vi "REV2mDistanceSensorRefNum Registry Set.vi"(8 "error in (no error)":errorcluster, 9 "Test Mode Only":bool, 10 "refnum name":string="REV2m", 11 "REV2mDistanceSensorsArray":T1={"Automatic Enabled"=TRUE, "Sensors[]"=[]}) -> (0 "error out":errorcluster, 3 "REV2mDistanceSensorsArray Out":T1={"Automatic Enabled"=TRUE, "Sensors[]"=[]})   [LabVIEW 2019, in "DistanceSensorDriver.lvlib"]
uses:
  DistanceSensorDriver.lvlib
  Typedef/Rev2mDistanceSensorsArray.ctl
  Typedef/REV2mDistanceSensorDevRef.ctl
  Typedef/Ports.ctl
  <vilib>/Rock Robotics/WPI/Utilities/Refnum Registry Operation.ctl
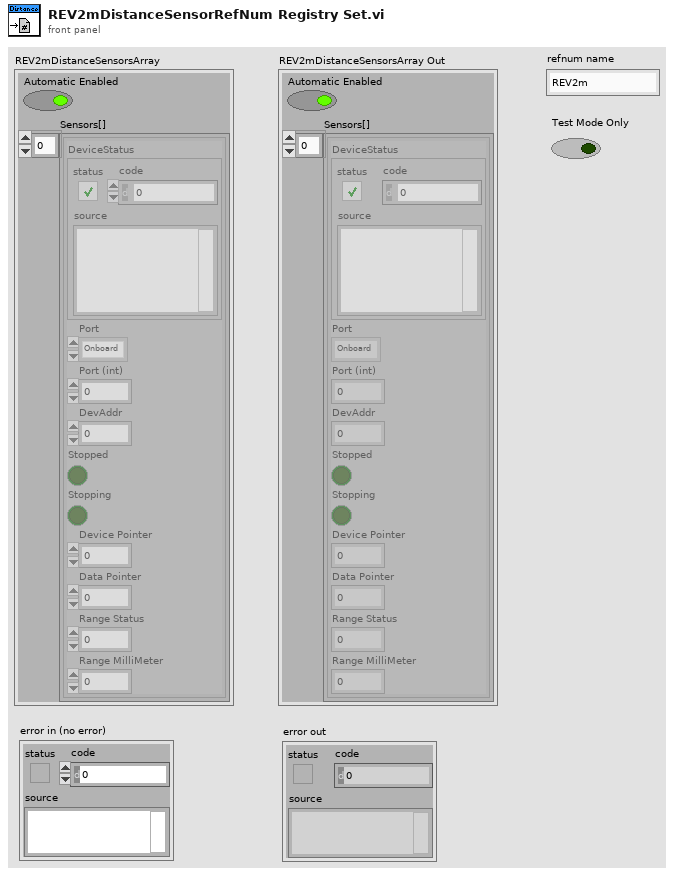
[diagram p1: front panel]
types:
  T1 = typedef "DistanceSensorDriver.lvlib/Rev2mDistanceSensorsArray.ctl" = cluster{"Automatic Enabled":bool, "Sensors[]":T2[]}
  T2 = typedef "DistanceSensorDriver.lvlib/REV2mDistanceSensorDevRef.ctl" = cluster{"DeviceStatus":errorcluster, "Port":T3, "Port (int)":i32, "DevAddr":i32, "Stopped":bool, "Stopping":bool, "Device Pointer":u64, "Data Pointer":u64, "Range Status":u8, "Range MilliMeter":u16}
  T3 = typedef "DistanceSensorDriver.lvlib/Ports.ctl" = enum32{"Onboard", "MXP"}
  T4 = typedef "Refnum Registry Operation.ctl" = enum16{"set", "get", "delete", "get all names", "read name"}
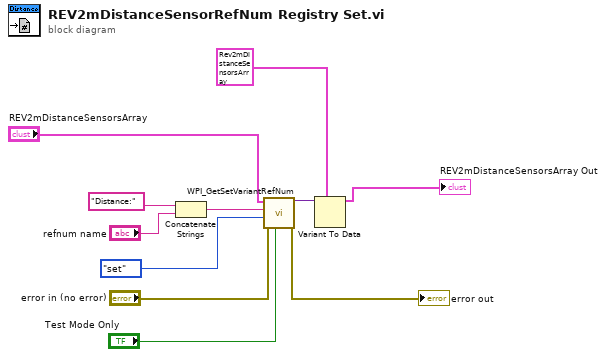
[diagram p0: block diagram]
diagram:
  n1 = Concatenate Strings("Distance:", "refnum name") -> (w11:string)
  n2 = call <vilib>:"WPI_GetSetVariantRefNum.vi"("Test Mode Only"="Test Mode Only", "error in (no error)"="error in (no error)", "Operation"=Refnum_Registry_Operation."set" ("menu"), "refnum name"=w11, "DevRef"="REV2mDistanceSensorsArray") -> ("error out"=→"error out":errorcluster, "DevRef"=w9:variant)  [unwired: 4 in, 1 out]
  n3 = Variant To Data(type=T1 {"Automatic Enabled"=FALSE, "Sensors[]"=[{"DeviceStatus"={"status"=TRUE, "code"=-1, "source"="DistanceSensorDriver.lvlib:VL53L0X_PerformRefSpadManagement.vi<ERR>\nRef Spad Management Error"}, "Port"=enum."Onboard", "Port (int)"=0, "DevAddr"=0, "Stopped"=FALSE, "Stopping"=FALSE, "Device Pointer"=0, "Data Pointer"=0, "Range Status"=0, "Range MilliMeter"=0}]} ("REV2mDistanceSensorsArray 3"), Variant=w9) -> (data=→"REV2mDistanceSensorsArray Out":T1)  [unwired: 1 in, 1 out]
